vi "JL_TS_Global_ERD_List.vi"(8 "Error In":errorcluster, 9 "Action":enum16{"Set", "Get "}(ring), 10 "ERD Numbers":u16[](array[numeric]), 11 "ERD Names":string[](array[string])) -> (0 "Error Out":errorcluster, 3 "TS ERD Names Number":T1)   [LabVIEW 2016]
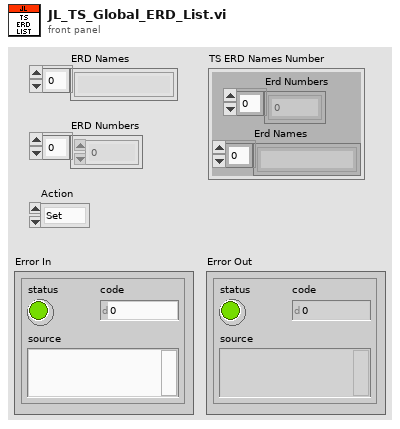
[diagram p1: front panel]
types:
  T1 = cluster{"Erd Numbers":u16[], "Erd Names":string[]}
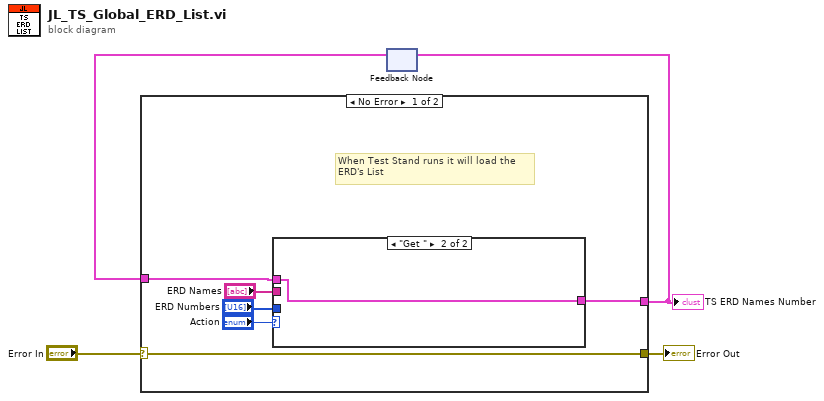
[diagram p0: block diagram]
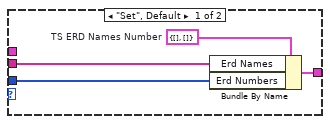
[diagram p2: hidden frame]
diagram:
  n1 = feedback #1() -> (w3:T1)  [unwired: 1 in]
  n2 = case shown="No Error" "Error In" {
    selector: "Error In" -> [w5 w16]
    tunnel: [w7 w17] -> w4
    tunnel: w3 -> [w6 w17]
    tunnel: [w5 w16] -> w1
    frame No Error {
      # "When Test Stand runs it will load the \nERD's List"
      n3 = case shown="\"Get \"" "Action" {
        tunnel: "ERD Names" -> [w14 _]
        tunnel: "ERD Numbers" -> [w13 _]
        tunnel: [w12 w15] -> w7
        tunnel: w6 -> [_ w15]
        frame "Set", Default {
          w11 = T1 {"Erd Numbers"=[], "Erd Names"=[]}  # TS ERD Names Number
          n4 = Bundle By Name(cluster=w11, "Erd Names"=w14, "Erd Numbers"=w13) -> (w12:T1)
        }
        frame "Get " {
        }
      }
    }
    frame Error {
    }
  }
  "TS ERD Names Number" <- w4
  "Error Out" <- w1
  n5 = feedback-in #1(w4) -> ()
